vi "Text_Hamming_test.vi"() -> ()   [LabVIEW 2014]
uses:
  <vilib>/addons/Modulation/Digital/Channel Coding/MT Hamming Encoder (Systematic).vi
  <vilib>/addons/Modulation/Digital/Channel Coding/MT Hamming Decoder (Systematic).vi
  <vilib>/addons/Modulation/niDMT.lvlib
panel:
  out "string":string
  out "message bitstream":i8[](array[numeric])
  out "Number of Packets":i32
  in  "Packet\nMessage Length (bits)":i32
  in  "text":string
  out "output bit stream 2":i8[](array[numeric]) caption="output bit stream"
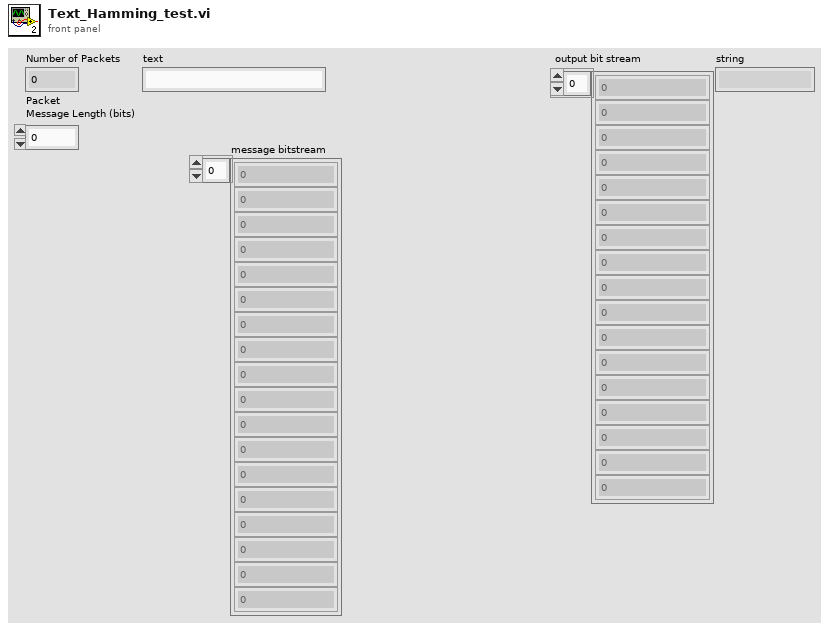
[diagram p1: front panel]
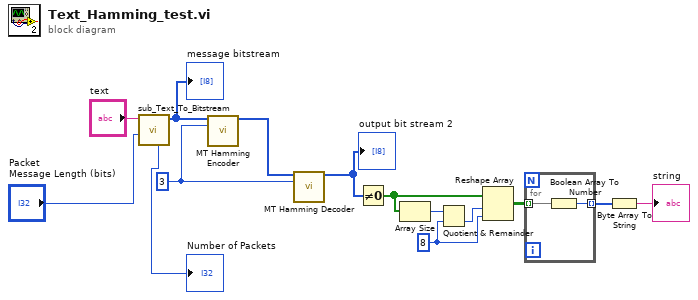
[diagram p0: block diagram]
diagram:
  w3 = 8
  w13 = 3 ("hamming order")
  n1 = call "sub_Text_To_Bitstream.vi"("Packet\nMessage Length (bits)"="Packet\nMessage Length (bits)", "text"="text") -> ("message bitstream"=w11:i8[], "Number of Packets"=→"Number of Packets":i32)  [unwired: 7 in, 1 out]
  "message bitstream" <- w11
  n2 = call-poly <vilib>:"MT Hamming Encoder.vi"("input bit stream"=w11, "hamming order"=w13) -> ("output bit stream"=w14:i8[])  [unwired: 12 in, 1 out]
  n3 = call-poly <vilib>:"MT Hamming Decoder.vi"("input bit stream"=w14, "hamming order"=w13) -> ("output bit stream"=w8:i8[])  [unwired: 12 in, 1 out]
  "output bit stream 2" <- w8
  n4 = Not Equal To 0?(x=w8) -> (x != 0?=w6:bool[])
  n5 = Array Size(array=w6) -> (size(s)=w4:i32)
  n6 = Quotient & Remainder(x=w4, y=w3) -> (floor(x/y)=w2:i32)  [unwired: 1 out]
  n7 = Reshape Array(w6, w2, w3) -> (w5:bool[][])
  n8 = for {
    tunnel: [w16] -> w7 mode=indexing
    tunnel: w5 -> [w15] mode=indexing
    n9 = Boolean Array To Number(Boolean array=w15) -> (number=w16:u32)
  }
  n10 = Byte Array To String(unsigned byte array=w7) -> (string=→"string":string)
